vi "Add UI Actor Event.vi"(8 "error in (no error)":errorcluster, 10 "Indicator Refnum":refnum<vi>) -> (0 "error out":errorcluster)   [LabVIEW 2020]
doc: "This vi takes an indicator on the Actor Core VI front panel and creates an associated user event for the actor. It creates the reference in Prelaunch Init, stores it in the class private data, closes it in Stop Core, and then creates a new event case in Actor Core and moves the indicator into the event case and wires it up."
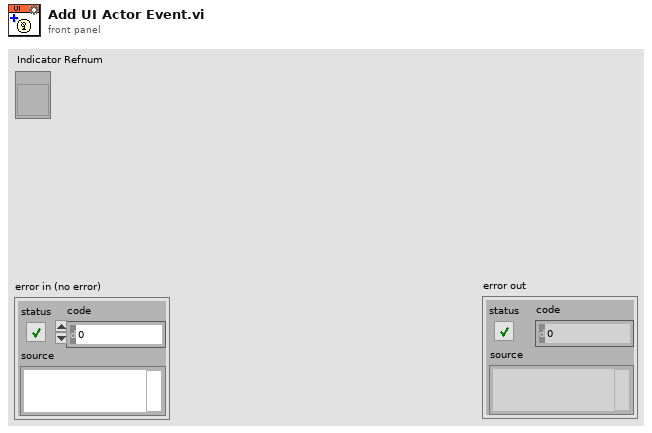
[diagram p1: front panel]
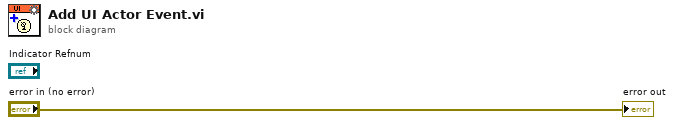
[diagram p0: block diagram]
diagram:
  "error out" <- "error in (no error)"
